vi "Get Scope Mode.vi"(8 "error in (no error)":errorcluster, 11 "VISA resource name":refnum<visa-resource-name>) -> (0 "error out":errorcluster, 2 "Scope Mode":i32, 3 "VISA resource name out":refnum<visa-resource-name>)   [LabVIEW 2013, in "Fluke 5XXX Series Multicalibrators.lvlib"]
doc: "This VI returns the oscilloscope’s current mode of operation.\n\nNote:\n\nThis VI is available only for instrument models 5500A and 5520A with oscilloscope option SC300 (SC600 or SC1100)."
uses:
  Fluke 5XXX Series Multicalibrators.lvlib
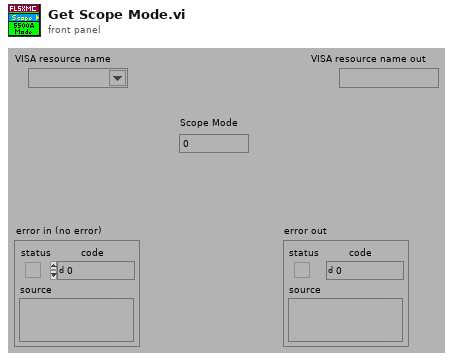
[diagram p1: front panel]
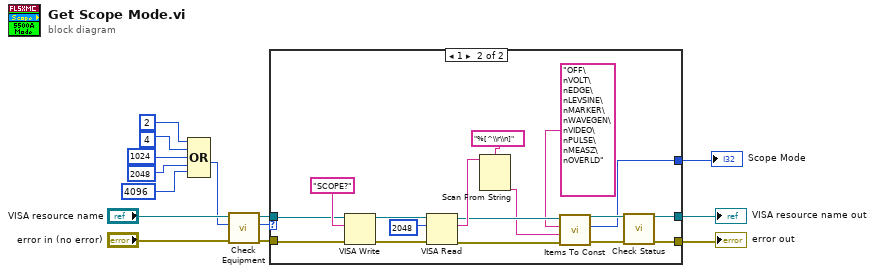
[diagram p0: block diagram]
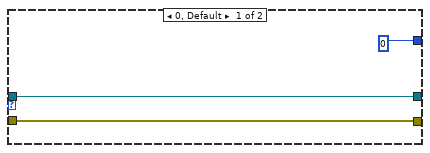
[diagram p2: hidden frame]
diagram:
  n1 = Compound Arithmetic op=OR(2 ("Numeric"), 4 ("Numeric"), 1024 ("Numeric"), 2048 ("Numeric"), 4096 ("Numeric")) -> (w1:i32)
  n2 = call "Check Equipment.vi"("error in (no error)"="error in (no error)", "Bit Mask"=w1, "VISA resource name"="VISA resource name") -> ("error out"=w14:errorcluster, "Present?"=w13:u32, "VISA resource name out"=w12:refnum<visa-resource-name>)  [unwired: 6 in]
  n3 = case shown="1" w13 {
    tunnel: [w17 w28] -> w9
    tunnel: [w16 w27] -> w8
    tunnel: w14 -> [w17 w30]
    tunnel: w12 -> [w16 w29]
    tunnel: [0 w19] -> w7
    frame 0, Default {
    }
    frame 1 {
      n4 = VISA Write(VISA resource name=w29, write buffer="SCOPE?", error in (no error)=w30) -> (VISA resource name out=w33:refnum<visa-resource-name>, error out=w32:errorcluster)  [unwired: 1 out]
      n5 = VISA Read(VISA resource name=w33, byte count=u32 2048 ("byte count (0)"), error in (no error)=w32) -> (VISA resource name out=w21:refnum<visa-resource-name>, read buffer=w25:string, error out=w22:errorcluster)  [unwired: 1 out]
      n6 = Scan From String(format string="%[^\\r\\n]", input string=w25) -> (output 1=w20:string)  [unwired: 3 in, 3 out]
      n7 = call "Items To Const.vi"("error in (no error)"=w22, "String Item"=w20, "Multi-Line String"="OFF\nVOLT\nEDGE\nLEVSINE\nMARKER\nWAVEGEN\nVIDEO\nPULSE\nMEASZ\nOVERLD", "VISA resource name"=w21) -> ("error out"=w23:errorcluster, "Index"=w19:i32, "VISA resource name out"=w24:refnum<visa-resource-name>)  [unwired: 5 in]
      n8 = call "Check Status.vi"("VISA resource name"=w24, "error in (no error)"=w23) -> ("VISA resource name out"=w27:refnum<visa-resource-name>, "error out"=w28:errorcluster)  [unwired: 12 in]
    }
  }
  "Scope Mode" <- w7
  "VISA resource name out" <- w8
  "error out" <- w9
